vi "hmi_knob.vi"(6 "configuration":T1={"dialog_text"="", "boolean_text_1"="", "boolean_text_2"="", "boolean_text_3"="", "inner_color"=16711680, "outer_color"=6618880, "wait_s"=nan, "error_status"=FALSE, "error_source"="", "error_details"="", "string []"=[], "custom_entry"=FALSE}, 7 "hmi_references":T2, 8 "error in (no error)":errorcluster, 10 "value_2 in":dbl, 11 "value_1 in":dbl) -> (0 "error out":errorcluster, 2 "value_2 out":dbl, 3 "value_1 out":dbl)   [LabVIEW 2015, in "lv-dialog-interfaces.lvlib"]
uses:
  lv-dialog-interfaces.lvlib
  _controls/hmi_references.ctl
  _controls/configuration.ctl
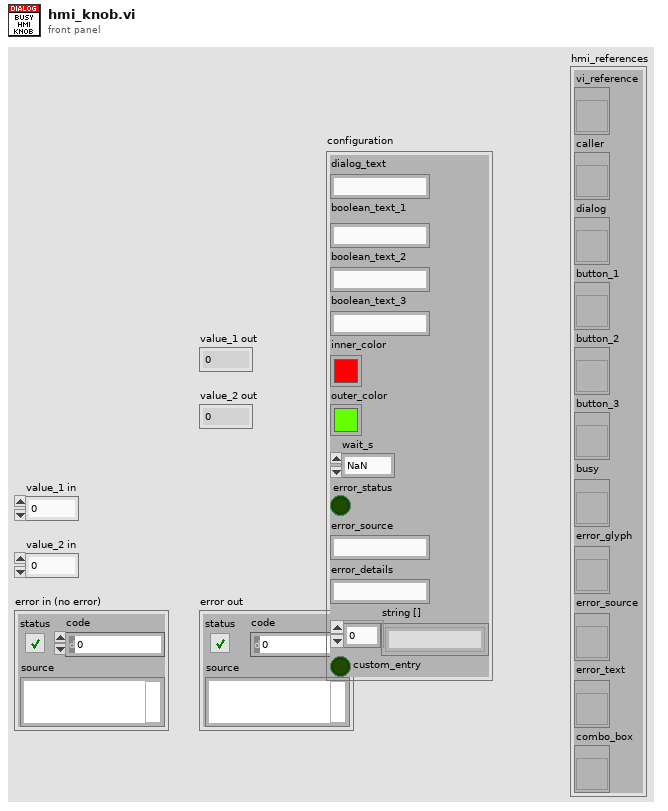
[diagram p1: front panel]
types:
  T1 = typedef "lv-dialog-interfaces.lvlib/configuration.ctl" = cluster{"dialog_text":string, "boolean_text_1":string, "boolean_text_2":string, "boolean_text_3":string, "inner_color":u32, "outer_color":u32, "wait_s":dbl, "error_status":bool, "error_source":string, "error_details":string, "string []":string[], "custom_entry":bool}
  T2 = typedef "lv-dialog-interfaces.lvlib/hmi_references.ctl" = cluster{"vi_reference":refnum<vi>, "caller":refnum<vi>, "dialog":refnum<vi>, "button_1":refnum<vi>, "button_2":refnum<vi>, "button_3":refnum<vi>, "busy":refnum<vi>, "error_glyph":refnum<vi>, "error_source":refnum<vi>, "error_text":refnum<vi>, "combo_box":refnum<vi>}
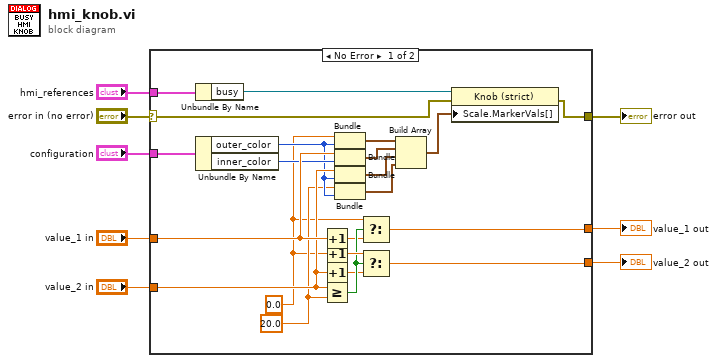
[diagram p0: block diagram]
diagram:
  n1 = case shown="No Error" "error in (no error)" {
    selector: "error in (no error)" -> [w29 w31]
    tunnel: [w30 w31] -> w8
    tunnel: "value_1 in" -> [w27 _]
    tunnel: "value_2 in" -> [w26 _]
    tunnel: [w22 _] -> w4
    tunnel: [w21 _] -> w3
    tunnel: "hmi_references" -> [w13 _]
    tunnel: "configuration" -> [w12 _]
    frame No Error {
      w10 = 20.0 ("maximum")
      w9 = 0.0 ("minimum")
      n2 = Unbundle By Name(w13) -> ("busy"=w15:refnum<vi>)
      n3 = Unbundle By Name(w12) -> ("outer_color"=w11:u32, "inner_color"=w14:u32)
      n4 = Increment(x=w27) -> (x+1=w23:dbl)
      n5 = Increment(x=w9) -> (x+1=w28:dbl)
      n6 = Increment(x=w26) -> (x+1=w24:dbl)
      n7 = Greater Or Equal?(x=w26, y=w10) -> (x >= y?=w25:bool)
      n8 = Bundle("minimum"=w9, "outer_color"=w11) -> (w18:cluster{"minimum":dbl, "outer_color":u32})  [unwired: 1 in]
      n9 = Bundle("value_1 in"=w27, "inner_color"=w14) -> (w20:cluster{"value_1 in":dbl, "inner_color":u32})  [unwired: 1 in]
      n10 = Bundle("value_2 in"=w26, "outer_color"=w11) -> (w17:cluster{"value_2 in":dbl, "outer_color":u32})  [unwired: 1 in]
      n11 = Bundle("maximum"=w10, "outer_color"=w11) -> (w16:cluster{"maximum":dbl, "outer_color":u32})  [unwired: 1 in]
      n12 = Select(t=w9, s=w25, f=w23) -> (s? t:f=w21:dbl)
      n13 = Select(t=w28, s=w25, f=w24) -> (s? t:f=w22:dbl)
      n14 = Build Array(w18, w20, w17, w16) -> (w19:cluster{"maximum":dbl, "outer_color":u32}[])
      n15 = property on="Property Node" class="Knob (strict)"(reference=w15, error in=w29, "Scale.MarkerVals[]"=w19) -> (error out=w30:errorcluster)  [unwired: 1 out]
    }
    frame Error {
    }
  }
  "error out" <- w8
  "value_2 out" <- w4
  "value_1 out" <- w3
